vi "Tosca-Start External Recording.vi"(0 "Connect":T3={"Tracking"=FALSE, "Synapse"=FALSE, "Pupil"=FALSE, "Loco"=FALSE, "Retrieve"=TRUE, "Codes"=""}, 5 "IPC":T2, 7 "Path":path=path "C:/Data/Tosca/Data/XYZ999/Session 6/XYZ999-Session6-Run19.txt", 11 "error in (no error)":errorcluster, 12 "AI":T1) -> (15 "error out":errorcluster={"status"=TRUE, "code"=54, "source"="TCP Open Connection in TCP-Send Command.vi:340001->Tosca-Start Synapse Recording.vi->Tosca-Start External Recording.vi->Tosca-Init Data Analysis.vi->Tosca.vi"})   [LabVIEW 2020]
uses:
  Classes/Parameters/Connect.ctl
  IPC VIs/Tosca-IPC.ctl
  Classes/Parameters/Parameters.lvclass
  Digital Input VIs/Tosca-DI Queue Data.ctl
  Digital Input VIs/Tosca-Input Event.ctl
  Digital Input VIs/Tosca-Input Criterion.ctl
  epl-vi-lib/Utility VIs/Type Defs/Logic State.ctl
  Typedefs/Tosca-Accumulator.ctl
  Typedefs/Tosca-State AODO.ctl
  Typedefs/Tosca-AO Runtime.ctl
  Typedefs/Tosca-DO Runtime.ctl
  epl-vi-lib/Signal Synthesis VIs/4th Generation/Classes/SignalManager/SignalManager.lvclass
  Typedefs/Tosca-Synapse Start Data.ctl
  IPC VIs/Tosca-Message.ctl
  IPC VIs/Tosca-Message Action.ctl
  Typedefs/Tosca-Thread Type.ctl
  Imaging VIs/Tosca-2P-Notifier Data.ctl
  Typedefs/Tosca-MATLAB Queue Data.ctl
  Visual Stim VIs/Tosca-Grating.ctl
  Visual Stim VIs/Tosca-Grating Type.ctl
  Typedefs/Tosca-File IO Notification.ctl
  Typedefs/Tosca-AI.ctl
  Typedefs/Tosca-Pupillometry Mode.ctl
panel:
  in  "Tracking":u16(ring)=1 caption="Tracking ready"
  in  "AI":u16(ring)=1 caption="Analog Input initializing..."
  in  "Loco":u16(ring) caption="Locomotion initializing..."
  in  "Pupil":u16(ring)=2 caption="Pupillometry initializing..."
  in  "Synapse":u16(ring)=1 caption="Synapse initializing..."
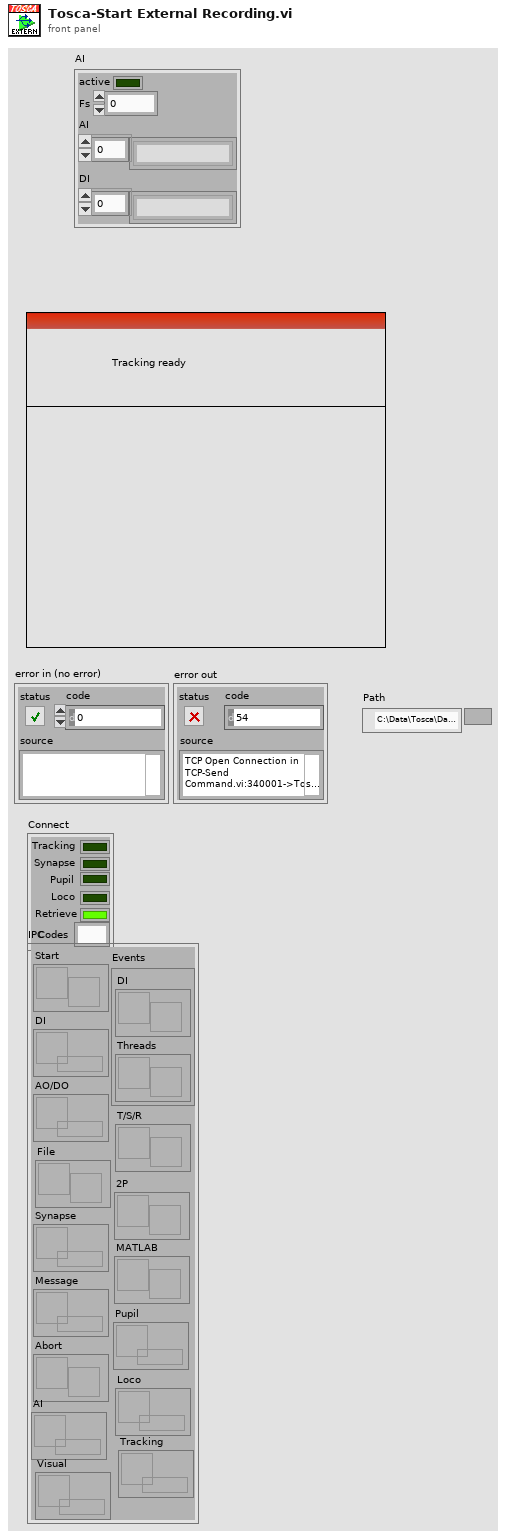
[diagram p1: front panel]
types:
  T1 = typedef "Tosca-AI.ctl" = cluster{"active":bool, "Fs":dbl, "AI":string[], "DI":string[]}
  T2 = typedef "Tosca-IPC.ctl" = cluster{"Start":refnum<notifier>, "DI":refnum<queue>, "AO/DO":refnum<queue>, "Synapse":refnum<queue>, "Message":refnum<queue>, "Abort":refnum<notifier>, "Events":cluster{"DI":refnum<user-event>, "Threads ":refnum<user-event>}, "T/S/R":refnum<notifier>, "2P":refnum<notifier>, "MATLAB":refnum<notifier>, "Pupil":refnum<queue>, "Loco":refnum<queue>, "AI":refnum<queue>, "Tracking":refnum<queue>, "Visual":refnum<queue>, "File":refnum<notifier>}
  T3 = typedef "Parameters.lvclass/Connect.ctl" = cluster{"Tracking":bool, "Synapse":bool, "Pupil":bool, "Loco":bool, "Retrieve":bool, "Codes":string}
  T4 = typedef "Tosca-Pupillometry Mode.ctl" = enum16{"OFF", "EPL", "ETMobile"}
  T5 = cluster{"Path out":path, "Codes":string, "Retrieve":bool}
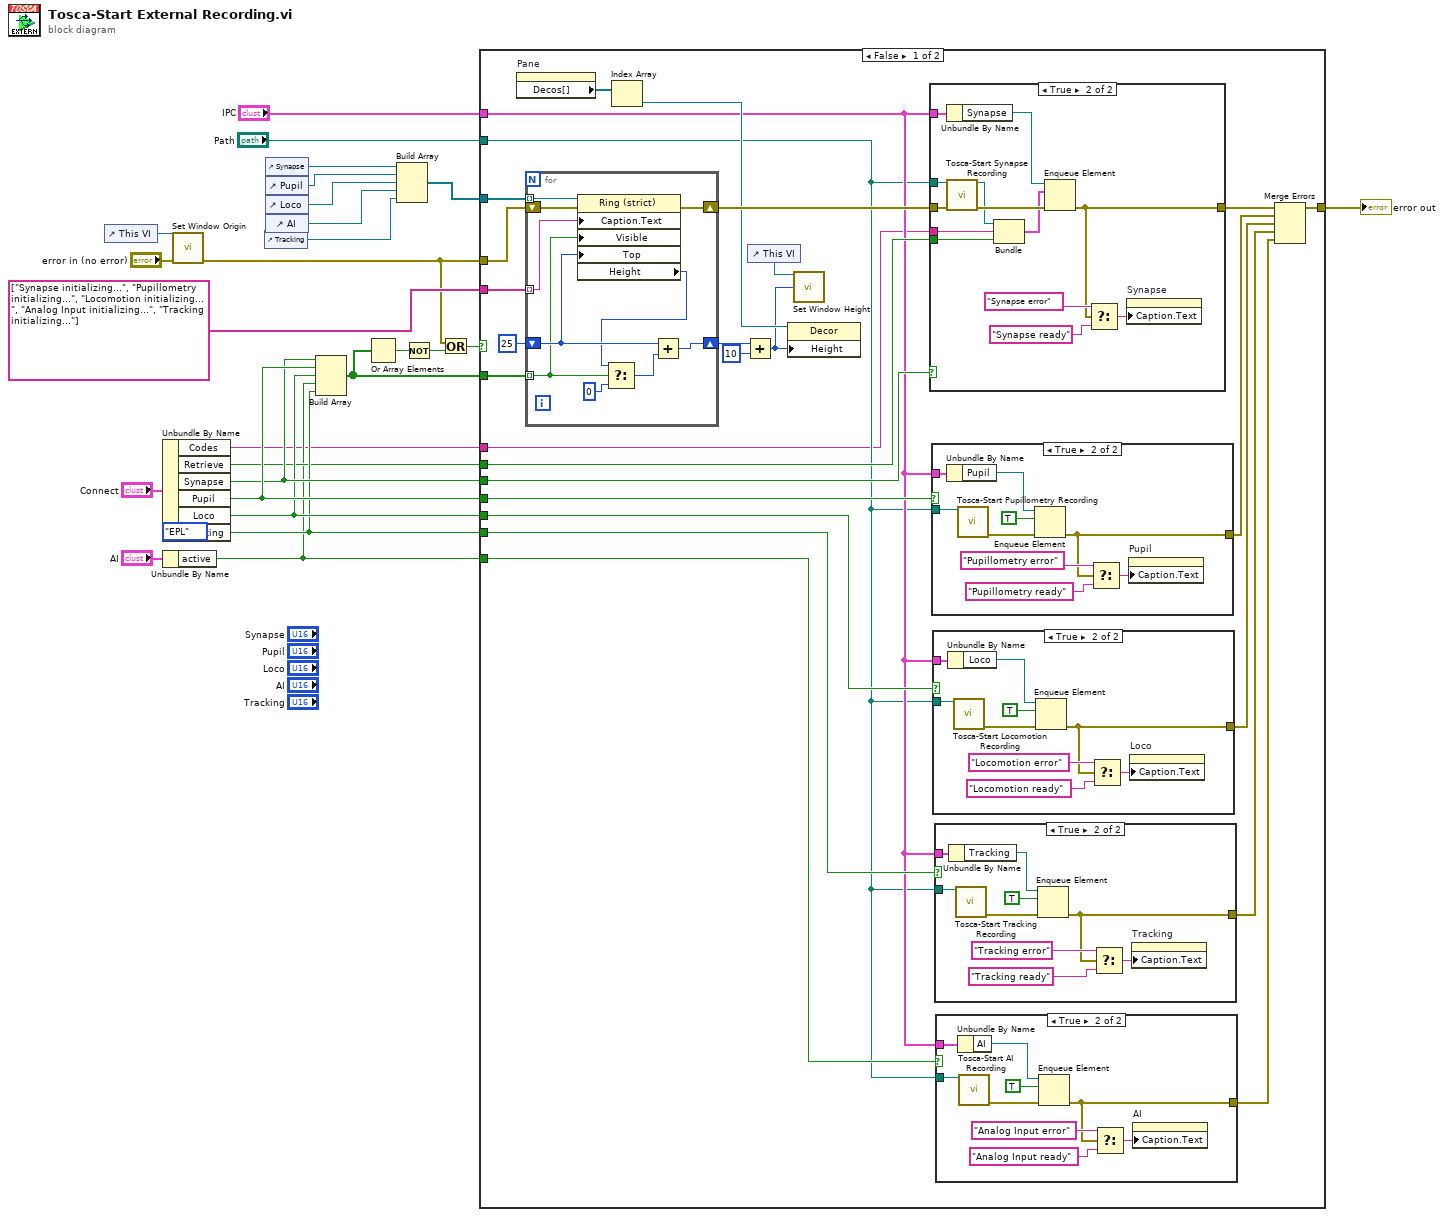
[diagram p0: block diagram]
diagram:
  (unwired) Tosca-Pupillometry_Mode."EPL" ("y")
  n1 = control-ref of="This VI"() -> (w9:refnum<vi>)
  n2 = Unbundle By Name("Connect") -> ("Codes"=w1:string, "Retrieve"=w3:bool, "Synapse"=w18:bool, "Pupil"=w25:bool, "Loco"=w8:bool, "Tracking"=w4:bool)
  n3 = Unbundle By Name("AI") -> ("active"=w2:bool)
  n4 = call "Set Window Origin.vi"("VI in"=w9, "error in (no error)"="error in (no error)") -> ("error out"=w10:errorcluster)  [unwired: 11 in, 2 out]
  n5 = control-ref of="Tracking"() -> (w5:refnum<vi>)
  n6 = control-ref of="Synapse"() -> (w15:refnum<vi>)
  n7 = control-ref of="Pupil"() -> (w14:refnum<vi>)
  n8 = control-ref of="Loco"() -> (w12:refnum<vi>)
  n9 = control-ref of="AI"() -> (w7:refnum<vi>)
  n10 = Build Array(w18, w25, w8, w2, w4) -> (w22:bool[])
  n11 = Or Array Elements(Boolean array=w22) -> (logical OR=w23:bool)
  n12 = Build Array(w15, w14, w12, w7, w5) -> (w24:refnum<vi>[])
  n13 = Not(x=w23) -> (.not. x?=w21:bool)
  n14 = Or(x=w10, y=w21) -> (x .or. y?=w20:bool)
  n15 = case shown="False" w20 {
    tunnel: w24 -> [w53 _]
    tunnel: w10 -> [w52 w114]
    tunnel: w22 -> [w51 _]
    tunnel: [w39 w114] -> w19
    tunnel: w18 -> [w49 _]
    tunnel: w25 -> [w37 _]
    tunnel: "Path" -> [w28 _]
    tunnel: "IPC" -> [w30 _]
    tunnel: string[] ["Synapse initializing...", "Pupillometry initializing...", "Locomotion initializing...", "Analog Input initializing...", "Tracking initializing..."] -> [w46 _]
    tunnel: w8 -> [w36 _]
    tunnel: w4 -> [w34 _]
    tunnel: w3 -> [w32 _]
    tunnel: w2 -> [w31 _]
    tunnel: w1 -> [w27 _]
    frame False {
      n16 = property on="Pane" class="Pane"() -> ("Decos[]"=w44:refnum<vi>[])  [unwired: 2 in, 2 out]
      n17 = for {
        tunnel: w53 -> [w86] mode=indexing
        shift-right: [w84] -> w48
        shift-left: w52 -> [w85]
        tunnel: w51 -> [w79] mode=indexing
        shift-right: [w82] -> w45
        shift-left: 25 -> [w83]
        tunnel: w46 -> [w78] mode=indexing
        n18 = property class="Ring (strict)"(reference=w86, error in=w85, "Caption.Text"=w78, "Visible"=w79, "Top"=w83) -> (error out=w84:errorcluster, "Height"=w77:u32)  [unwired: 1 out]
        n19 = Select(t=w77, s=w79, f=0) -> (s? t:f=w81:u32)
        n20 = Add(x=w83, y=w81) -> (x+y=w82:u32)
      }
      n21 = Index Array(array=w44) -> (element=w43:refnum<vi>)  [unwired: 1 in]
      n22 = Add(x=w45, y=10) -> (x+y=w41:u32)
      n23 = control-ref of="This VI"() -> (w40:refnum<vi>)
      n24 = property class="Decor"(reference=w43, "Height"=w41) -> ()  [unwired: 1 in, 2 out]
      n25 = call "Set Window Height.vi"("VI in"=w40, "Height"=w41) -> ()  [unwired: 12 in, 2 out]
      n26 = case shown="True" w49 {
        tunnel: w48 -> [w63 w76]
        tunnel: [w63 w69] -> w47
        tunnel: w28 -> [_ w75]
        tunnel: w30 -> [_ w74]
        tunnel: w32 -> [_ w65]
        tunnel: w27 -> [_ w64]
        frame False {
        }
        frame True {
          n27 = Unbundle By Name(w74) -> ("Synapse"=w73:refnum<queue>)
          n28 = call "Tosca-Start Synapse Recording.vi"("Path"=w75, "error in (no error)"=w76) -> ("Path out"=w67:path, "error out"=w72:errorcluster)  [unwired: 12 in]
          n29 = Bundle("Path out"=w67, "Codes"=w64, "Retrieve"=w65) -> (w66:T5)  [unwired: 1 in]
          n30 = Enqueue Element(queue=w73, element=w66, error in (no error)=w72) -> (error out=w69:errorcluster)  [unwired: 1 in, 2 out]
          n31 = Select(t="Synapse error", s=w69, f="Synapse ready") -> (s? t:f=w68:string)
          n32 = property on="Synapse" class="Ring (strict)"("Caption.Text"=w68) -> ()  [unwired: 2 in, 2 out]
        }
      }
      n33 = case shown="True" w37 {
        tunnel: [_ w56] -> w38
        tunnel: w30 -> [_ w62]
        tunnel: w28 -> [_ w54]
        frame False {
        }
        frame True {
          n34 = Unbundle By Name(w62) -> ("Pupil"=w61:refnum<queue>)
          n35 = call "Tosca-Start Pupillometry Recording.vi"("Path"=w54) -> ("error out"=w60:errorcluster)  [unwired: 14 in]
          n36 = Enqueue Element(queue=w61, element=TRUE, error in (no error)=w60) -> (error out=w56:errorcluster)  [unwired: 1 in, 2 out]
          n37 = Select(t="Pupillometry error", s=w56, f="Pupillometry ready") -> (s? t:f=w55:string)
          n38 = property on="Pupil" class="Ring (strict)"("Caption.Text"=w55) -> ()  [unwired: 2 in, 2 out]
        }
      }
      n39 = case shown="True" w36 {
        tunnel: [_ w90] -> w35
        tunnel: w30 -> [_ w95]
        tunnel: w28 -> [_ w88]
        frame False {
        }
        frame True {
          n40 = Unbundle By Name(w95) -> ("Loco"=w94:refnum<queue>)
          n41 = call "Tosca-Start Locomotion Recording.vi"("Path"=w88) -> ("error out"=w87:errorcluster)  [unwired: 14 in]
          n42 = Enqueue Element(queue=w94, element=TRUE, error in (no error)=w87) -> (error out=w90:errorcluster)  [unwired: 1 in, 2 out]
          n43 = Select(t="Locomotion error", s=w90, f="Locomotion ready") -> (s? t:f=w89:string)
          n44 = property on="Loco" class="Ring (strict)"("Caption.Text"=w89) -> ()  [unwired: 2 in, 2 out]
        }
      }
      n45 = case shown="True" w34 {
        tunnel: [_ w99] -> w33
        tunnel: w30 -> [_ w104]
        tunnel: w28 -> [_ w97]
        frame False {
        }
        frame True {
          n46 = Unbundle By Name(w104) -> ("Tracking"=w103:refnum<queue>)
          n47 = call "Tosca-Start Tracking Recording.vi"("Path"=w97) -> ("error out"=w96:errorcluster)  [unwired: 14 in]
          n48 = Enqueue Element(queue=w103, element=TRUE, error in (no error)=w96) -> (error out=w99:errorcluster)  [unwired: 1 in, 2 out]
          n49 = Select(t="Tracking error", s=w99, f="Tracking ready") -> (s? t:f=w98:string)
          n50 = property on="Tracking" class="Ring (strict)"("Caption.Text"=w98) -> ()  [unwired: 2 in, 2 out]
        }
      }
      n51 = case shown="True" w31 {
        tunnel: [_ w108] -> w29
        tunnel: w30 -> [_ w113]
        tunnel: w28 -> [_ w106]
        frame False {
        }
        frame True {
          n52 = Unbundle By Name(w113) -> ("AI"=w112:refnum<queue>)
          n53 = call "Tosca-Start AI Recording.vi"("Path"=w106) -> ("error out"=w105:errorcluster)  [unwired: 14 in]
          n54 = Enqueue Element(queue=w112, element=TRUE, error in (no error)=w105) -> (error out=w108:errorcluster)  [unwired: 1 in, 2 out]
          n55 = Select(t="Analog Input error", s=w108, f="Analog Input ready") -> (s? t:f=w107:string)
          n56 = property on="AI" class="Ring (strict)"("Caption.Text"=w107) -> ()  [unwired: 2 in, 2 out]
        }
      }
      n57 = Merge Errors(w47, w38, w35, w33, w29) -> (w39:errorcluster)
    }
    frame True {
    }
  }
  "error out" <- w19
